vi "RSZVB Trace Response Data All.vi"(8 "error in (no error)":errorcluster {"code" format="%.0x"}, 9 "Data Format (0: Unformatted)":i32(ring) items=["Unformatted", "Formatted", "Unformatted With Trace Mathematics"], 10 "Channel (Trace) (1)":i32=1, 11 "VISA session":refnum<visa-resource-name>) -> (0 "error out":errorcluster {"code" format="%.0x"}, 2 "Trace Data":dbl[](array[numeric]) format="%^.3e", 3 "dup VISA session":refnum<visa-resource-name>)   [LabVIEW 2011]
doc: "This VI reads the current response values of all traces of the current test setup.\n\nRemote-control command(s):\nFORMat[:DATA] REAL ,32\nCALCulate<Ch>:DATA:ALL? FDATa | SDATa | MDATa"
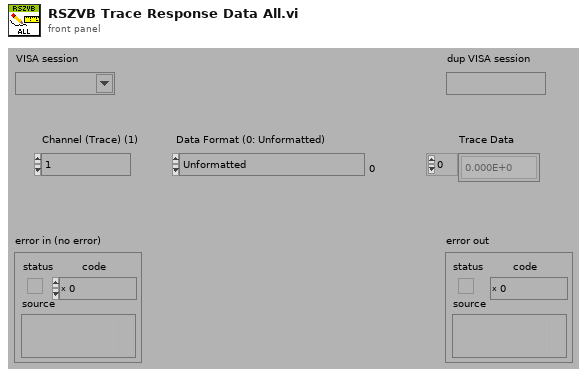
[diagram p1: front panel]
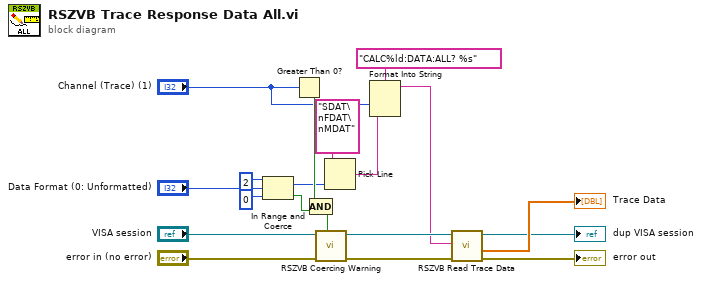
[diagram p0: block diagram]
diagram:
  n1 = In Range and Coerce(upper limit=2, x="Data Format (0: Unformatted)", lower limit=0) -> (coerced(x)=w11:i32, In Range?=w16:bool)
  n2 = Greater Than 0?(x="Channel (Trace) (1)") -> (x > 0?=w17:bool)
  n3 = Compound Arithmetic op=AND(w17, w16) -> (w18:bool)
  n4 = call "RSZVB Coercing Warning.vi"("In Range?"=w18, "error in (no error)"="error in (no error)", "VISA session"="VISA session") -> ("error out"=w15:errorcluster, "dup VISA session"=w14:refnum<visa-resource-name>)  [unwired: 7 in]
  n5 = Pick Line(multi-line string="SDAT\nFDAT\nMDAT", line index=w11) -> (output string=w9:string)  [unwired: 1 in]
  n6 = Format Into String(format string="CALC%ld:DATA:ALL? %s", "Channel (Trace) (1)", w9) -> (resulting string=w8:string)  [unwired: 2 in, 1 out]
  n7 = call "RSZVB Read Trace Data.vi"("error in (no error)"=w15, "Buffer"=w8, "VISA session"=w14) -> ("error out"=→"error out":errorcluster, "Trace Data"=→"Trace Data":dbl[], "dup VISA session"=→"dup VISA session":refnum<visa-resource-name>)  [unwired: 6 in]
